vi "charts-and-waveforms.vi"() -> ()   [LabVIEW 2025]
uses:
  <vilib>/measure/NI_MABase.lvlib
panel:
  in  "signal type":T1(ring)
  in  "signal":dbl(slide) scale=0.0..10.0
  out "Waveform Chart":waveform(dbl)(graph)
  out "Waveform Graph 2":dbl[](graph)
  in  "Array":dbl[](array[numeric])
  in  "freq":dbl
  in  "amp":dbl
  out "Waveform Graph":waveform(dbl)(graph)
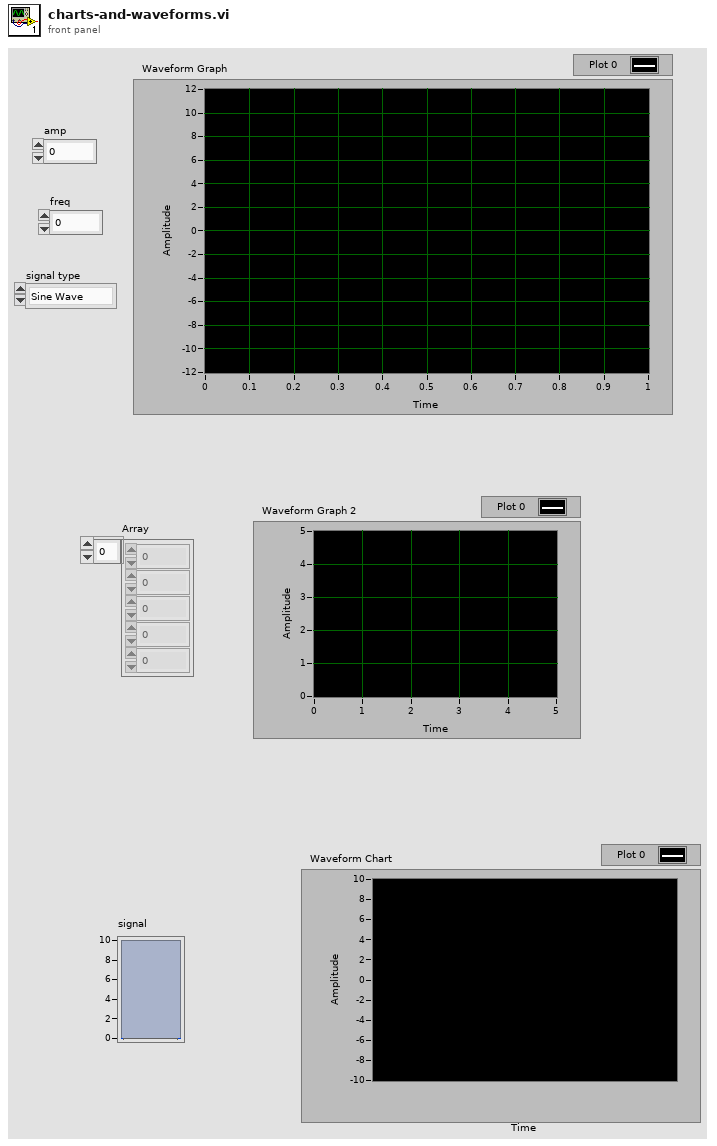
[diagram p1: front panel]
types:
  T1 = enum16{"Sine Wave", "Triangle Wave", "Square Wave", "Sawtooth Wave"}
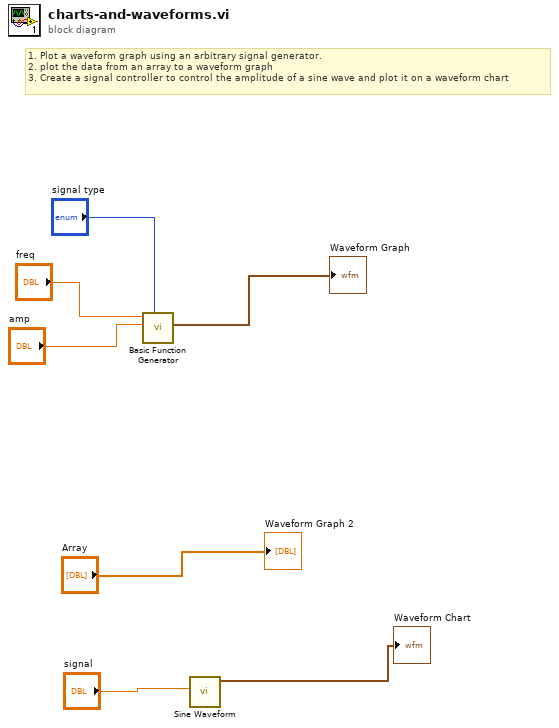
[diagram p0: block diagram]
diagram:
  # "1. Plot a waveform graph using an arbitrary signal generator. \n2. plot the data from an array to a waveform graph\n3. Create a signal controller to control the amplitude of a sine wave and plot it on a waveform chart"
  n1 = call <vilib>:"Basic Function Generator.vi"("signal type"="signal type", "amplitude"="amp", "frequency"="freq") -> ("signal out"=→"Waveform Graph":waveform(dbl))  [unwired: 6 in, 2 out]
  n2 = call <vilib>:"Sine Waveform.vi"("amplitude"="signal") -> ("signal out"=→"Waveform Chart":waveform(dbl))  [unwired: 9 in, 1 out]
  "Waveform Graph 2" <- "Array"
